vi "DSF.Engine.Framework.Initialize.Transfer Groups.Order by Priority.vi"(8 "error in (no error)":errorcluster, 10 "Transfer Groups":refnum<class "DSF.Engine.Transfer Group.lvclass">[](array[class]), 11 "Framework in":refnum<class "DSF.Engine.Framework.lvclass">) -> (0 "error out":errorcluster, 2 "sorted Transfer Groups":refnum<class "DSF.Engine.Transfer Group.lvclass">[](array[class]), 3 "Framework out":refnum<class "DSF.Engine.Framework.lvclass">)   [LabVIEW 2017, in "DSF.Engine.lvlib" / "DSF.Engine.Framework.lvclass"]
uses:
  DSF.Engine.Framework.lvclass
  Transfer/DSF.Engine.Transfer Group.lvclass
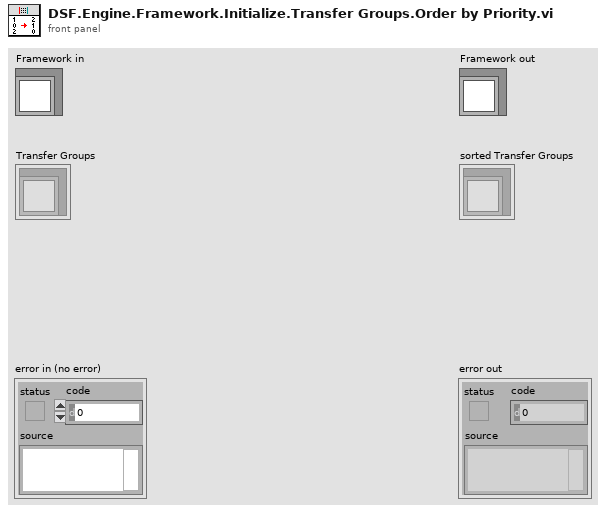
[diagram p1: front panel]
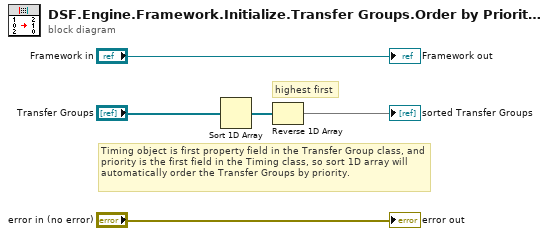
[diagram p0: block diagram]
diagram:
  # "highest first"
  # "Timing object is first property field in the Transfer Group class, and priority is the first field in the Timing class, so sort 1D array will automatically order the Transfer Groups by priority."
  n1 = Sort 1D Array(array="Transfer Groups") -> (sorted array=w4:refnum<class "DSF.Engine.Transfer Group.lvclass">[])
  n2 = Reverse 1D Array(array=w4) -> (reversed array=→"sorted Transfer Groups":refnum<class "DSF.Engine.Transfer Group.lvclass">[])
  "error out" <- "error in (no error)"
  "Framework out" <- "Framework in"
